vi "Collective state.vi"(11 "collective state":u8) -> (0 "error out":errorcluster, 2 "Warnings":errorcluster[](array[cluster]), 3 "Warning":bool)   [LabVIEW 2021, in "ELAN PDU.lvclass"]
uses:
  ELAN PDU.lvclass
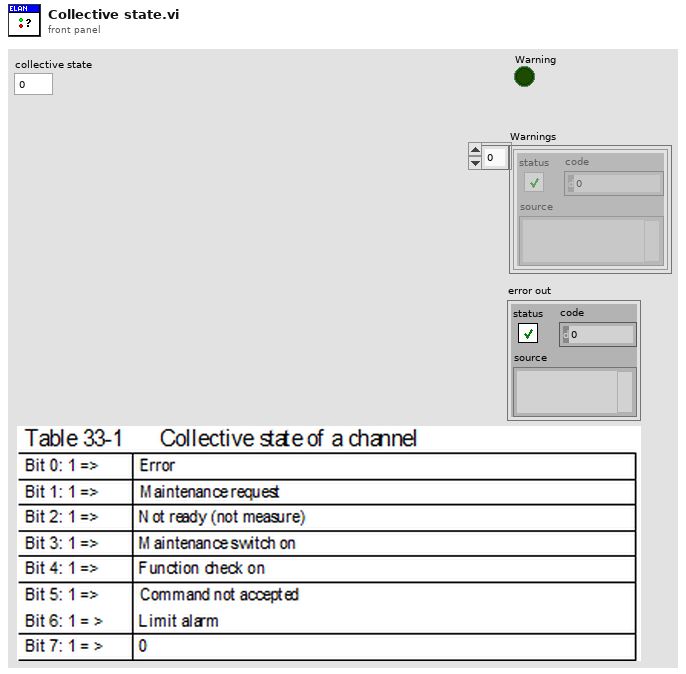
[diagram p1: front panel]
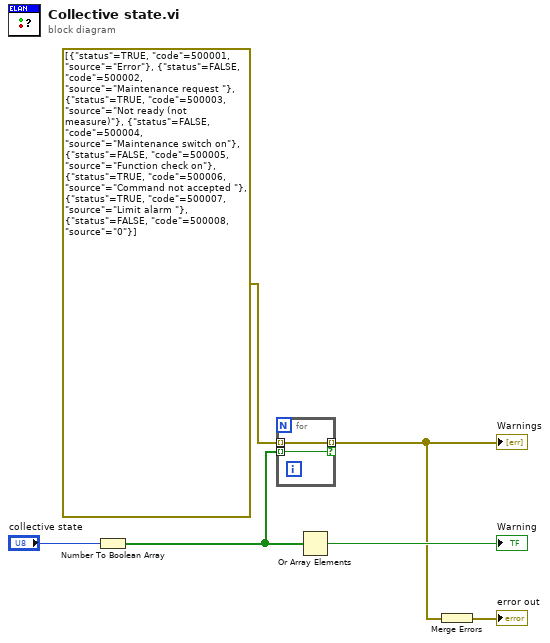
[diagram p0: block diagram]
diagram:
  n1 = Number To Boolean Array(number="collective state") -> (Boolean array=w5:bool[])
  n2 = for {
    tunnel: errorcluster[] [{"status"=TRUE, "code"=500001, "source"="Error"}, {"status"=FALSE, "code"=500002, "source"="Maintenance request "}, {"status"=TRUE, "code"=500003, "source"="Not ready (not measure)"}, {"status"=FALSE, "code"=500004, "source"="Maintenance switch on"}, {"status"=FALSE, "code"=500005, "source"="Function check on"}, {"status"=TRUE, "code"=500006, "source"="Command not accepted "}, {"status"=TRUE, "code"=500007, "source"="Limit alarm "}, {"status"=FALSE, "code"=500008, "source"="0"}] -> [w8] mode=indexing
    tunnel: w5 -> [w7] mode=indexing
    tunnel: [w8] -> w2 mode=indexing if=w7
  }
  "Warnings" <- w2
  n3 = Or Array Elements(Boolean array=w5) -> (logical OR=→"Warning":bool)
  n4 = Merge Errors(w2) -> (→"error out":errorcluster)
